vi "CTRE_CAN_GetTwoParam16.vi"(8 "error in (no error)":errorcluster, 11 "ArbID":u32) -> (0 "error out":errorcluster, 2 "2Params":u16[](array[numeric]), 3 "ArbID Out":u32)   [LabVIEW 2016]
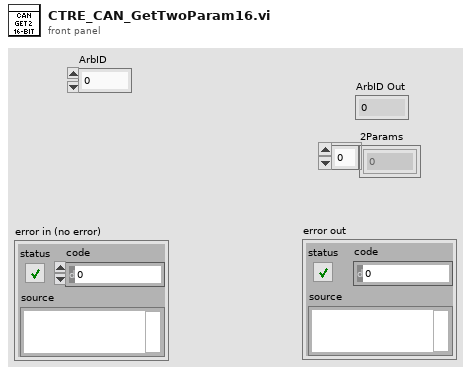
[diagram p1: front panel]
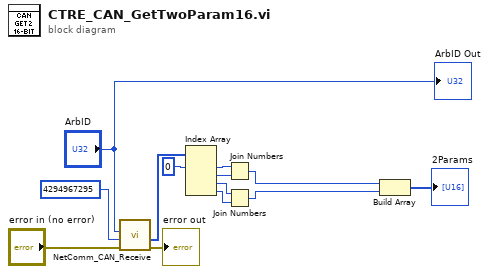
[diagram p0: block diagram]
diagram:
  n1 = call <vilib>:"NetComm_CAN_Receive.vi"("error in (no error)"="error in (no error)", "Message ID Mask"=u32 4294967295, "Message ID"="ArbID") -> ("error out"=→"error out":errorcluster, "Data"=w8:u8[])  [unwired: 5 in, 2 out]
  n2 = Index Array(array=w8, index #1=0 ("index")) -> (element #1=w9:u8, element #2=w10:u8, element #3=w11:u8, element #4=w12:u8)  [unwired: 3 in]
  n3 = Join Numbers(hi=w9, lo=w10) -> ((hi.lo)=w3:u16)
  n4 = Join Numbers(hi=w11, lo=w12) -> ((hi.lo)=w2:u16)
  n5 = Build Array(w3, w2) -> (→"2Params":u16[])
  "ArbID Out" <- "ArbID"
